vi "报警流程.vi"   [LabVIEW 2016, in "环境动力单元.lvlib"]
uses:
  <vilib>/ptbypt/NI_PtbyPt.lvlib
types:
  T1 = cluster{"低压报警阈值 V":dbl, "低压报警解除阈值 V":dbl, "高温报警阈值 ℃":dbl, "高温报警解除阈值 ℃":dbl, "湿度报警阈值 %":dbl, "湿度报警解除阈值 %":dbl}
  T2 = cluster{"蓄电池电压":dbl, "室温":dbl, "湿度":dbl, "水浸报警":bool, "烟雾报警":bool, "门禁状态":bool}
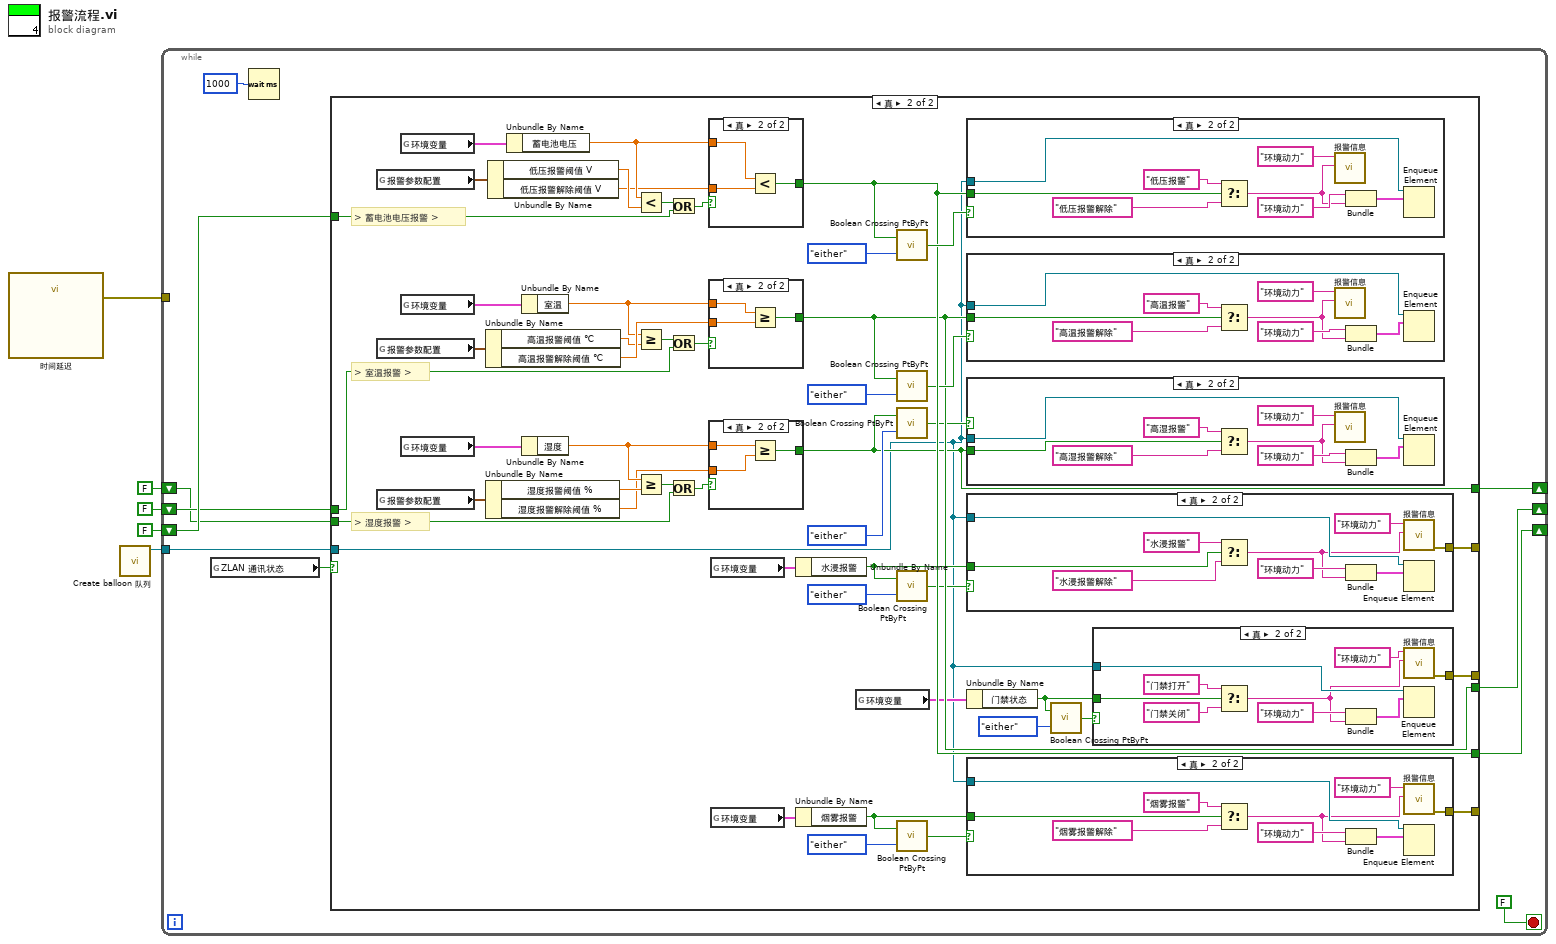
[diagram p0: block diagram]
diagram:
  n1 = call "时间延迟"() -> ("error out"=w1:errorcluster)  [unwired: 11 in]
  n2 = call "Create balloon 队列.vi"() -> ("队列输出"=w5:refnum<queue>)  [unwired: 11 in]
  n3 = while {
    shift-right: [w13] -> _
    shift-left: FALSE -> [w12]
    shift-right: [w10] -> _
    shift-left: FALSE -> [w11]
    shift-right: [w9] -> _
    shift-left: FALSE -> [w8]
    tunnel: w5 -> [w6]
    tunnel: w1 -> [_]
    stop <- FALSE stop-if-true
    n4 = global read "通讯全局变量.vi" "ZLAN 通讯状态"() -> (w7:bool)
    n5 = Wait (ms)(milliseconds to wait=u32 1000 ("等待时间（毫秒）")) -> ()  [unwired: 1 out]
    n6 = case shown="真" w7 {
      tunnel: [_ w38] -> w13
      tunnel: w12 -> [_ w57]
      tunnel: w11 -> [_ w56]
      tunnel: [_ w35] -> w10
      tunnel: [_ w32] -> w9
      tunnel: w8 -> [_ w41]
      tunnel: [_ w27] -> _
      tunnel: [_ w26] -> _
      tunnel: [_ w17] -> _
      tunnel: w6 -> [_ w16]
      frame False {
      }
      frame True {
        # "> 湿度报警 >"
        # "> 室温报警 >"
        # "> 蓄电池电压报警 >"
        n7 = global read "通讯全局变量断电保存.vi" "报警参数配置"() -> (w64:T1)
        n8 = global read "通讯全局变量断电保存.vi" "报警参数配置"() -> (w49:T1)
        n9 = global read "通讯全局变量断电保存.vi" "报警参数配置"() -> (w48:T1)
        n10 = global read "通讯全局变量.vi" "环境变量"() -> (w63:T2)
        n11 = global read "通讯全局变量.vi" "环境变量"() -> (w50:T2)
        n12 = global read "通讯全局变量.vi" "环境变量"() -> (w47:T2)
        n13 = Unbundle By Name(w49) -> ("高温报警阈值 ℃"=w51:dbl, "高温报警解除阈值 ℃"=w54:dbl)
        n14 = Unbundle By Name(w48) -> ("湿度报警阈值 %"=w46:dbl, "湿度报警解除阈值 %"=w43:dbl)
        n15 = Unbundle By Name(w64) -> ("低压报警阈值 V"=w62:dbl, "低压报警解除阈值 V"=w59:dbl)
        n16 = Unbundle By Name(w63) -> ("蓄电池电压"=w60:dbl)
        n17 = Unbundle By Name(w50) -> ("室温"=w53:dbl)
        n18 = Unbundle By Name(w47) -> ("湿度"=w44:dbl)
        n19 = Less?(x=w60, y=w62) -> (x < y?=w61:bool)
        n20 = Greater Or Equal?(x=w53, y=w51) -> (x >= y?=w52:bool)
        n21 = Greater Or Equal?(x=w44, y=w46) -> (x >= y?=w45:bool)
        n22 = Or(x=w61, y=w57) -> (x .or. y?=w58:bool)
        n23 = Or(x=w52, y=w56) -> (x .or. y?=w55:bool)
        n24 = Or(x=w45, y=w41) -> (x .or. y?=w42:bool)
        n25 = case shown="真" w58 {
          tunnel: w60 -> [_ w124]
          tunnel: w59 -> [_ w123]
          tunnel: [_ w122] -> w38
          frame False {
          }
          frame True {
            n26 = Less?(x=w124, y=w123) -> (x < y?=w122:bool)
          }
        }
        n27 = case shown="真" w55 {
          tunnel: w53 -> [_ w121]
          tunnel: w54 -> [_ w120]
          tunnel: [_ w119] -> w35
          frame False {
          }
          frame True {
            n28 = Greater Or Equal?(x=w121, y=w120) -> (x >= y?=w119:bool)
          }
        }
        n29 = case shown="真" w42 {
          tunnel: w44 -> [_ w118]
          tunnel: w43 -> [_ w117]
          tunnel: [_ w116] -> w32
          frame False {
          }
          frame True {
            n30 = Greater Or Equal?(x=w118, y=w117) -> (x >= y?=w116:bool)
          }
        }
        n31 = global read "通讯全局变量.vi" "环境变量"() -> (w29:T2)
        n32 = global read "通讯全局变量.vi" "环境变量"() -> (w24:T2)
        n33 = Unbundle By Name(w29) -> ("水浸报警"=w28:bool)
        n34 = Unbundle By Name(w24) -> ("烟雾报警"=w25:bool)
        n35 = global read "通讯全局变量.vi" "环境变量"() -> (w19:T2)
        n36 = call <vilib>:"Boolean Crossing PtByPt.vi"("direction"=enum16{"either", "false-true", "true-false"}."either", "input"=w38) -> ("crossing"=w39:bool)  [unwired: 1 in]
        n37 = call <vilib>:"Boolean Crossing PtByPt.vi"("direction"=enum16{"either", "false-true", "true-false"}."either", "input"=w35) -> ("crossing"=w36:bool)  [unwired: 1 in]
        n38 = call <vilib>:"Boolean Crossing PtByPt.vi"("direction"=enum16{"either", "false-true", "true-false"}."either", "input"=w32) -> ("crossing"=w34:bool)  [unwired: 1 in]
        n39 = call <vilib>:"Boolean Crossing PtByPt.vi"("direction"=enum16{"either", "false-true", "true-false"}."either", "input"=w28) -> ("crossing"=w30:bool)  [unwired: 1 in]
        n40 = call <vilib>:"Boolean Crossing PtByPt.vi"("direction"=enum16{"either", "false-true", "true-false"}."either", "input"=w25) -> ("crossing"=w23:bool)  [unwired: 1 in]
        n41 = case shown="真" w39 {
          tunnel: w38 -> [_ w114]
          tunnel: w16 -> [_ w109]
          frame False {
          }
          frame True {
            n42 = Select(t="低压报警" ("设备"), s=w114, f="低压报警解除" ("设备")) -> (s? t:f=w108:string)
            n43 = call "报警信息.vi"("报警信息"=w108, "设备"="环境动力") -> ()  [unwired: 9 in, 1 out]
            n44 = Bundle("设备"="环境动力", "设备"=w108) -> (w110:cluster{"设备":string, "设备":string})  [unwired: 1 in]
            n45 = Enqueue Element(queue=w109, element=w110) -> ()  [unwired: 2 in, 3 out]
          }
        }
        n46 = case shown="真" w36 {
          tunnel: w35 -> [_ w106]
          tunnel: w16 -> [_ w101]
          frame False {
          }
          frame True {
            n47 = Select(t="高温报警" ("设备"), s=w106, f="高温报警解除" ("设备")) -> (s? t:f=w100:string)
            n48 = call "报警信息.vi"("报警信息"=w100, "设备"="环境动力") -> ()  [unwired: 9 in, 1 out]
            n49 = Bundle("设备"="环境动力", "设备"=w100) -> (w102:cluster{"设备":string, "设备":string})  [unwired: 1 in]
            n50 = Enqueue Element(queue=w101, element=w102) -> ()  [unwired: 2 in, 3 out]
          }
        }
        n51 = case shown="真" w34 {
          tunnel: w32 -> [_ w98]
          tunnel: w16 -> [_ w93]
          frame False {
          }
          frame True {
            n52 = Select(t="高湿报警" ("设备"), s=w98, f="高湿报警解除" ("设备")) -> (s? t:f=w92:string)
            n53 = call "报警信息.vi"("报警信息"=w92, "设备"="环境动力") -> ()  [unwired: 9 in, 1 out]
            n54 = Bundle("设备"="环境动力", "设备"=w92) -> (w95:cluster{"设备":string, "设备":string})  [unwired: 1 in]
            n55 = Enqueue Element(queue=w93, element=w95) -> ()  [unwired: 2 in, 3 out]
          }
        }
        n56 = case shown="真" w30 {
          tunnel: w28 -> [_ w90]
          tunnel: [_ w87] -> w27
          tunnel: w16 -> [_ w84]
          frame False {
          }
          frame True {
            n57 = Select(t="水浸报警" ("设备"), s=w90, f="水浸报警解除" ("设备")) -> (s? t:f=w83:string)
            n58 = Bundle("设备"="环境动力", "设备"=w83) -> (w86:cluster{"设备":string, "设备":string})  [unwired: 1 in]
            n59 = call "报警信息.vi"("报警信息"=w83, "设备"="环境动力") -> ("error out"=w87:errorcluster)  [unwired: 9 in]
            n60 = Enqueue Element(queue=w84, element=w86) -> ()  [unwired: 2 in, 3 out]
          }
        }
        n61 = Unbundle By Name(w19) -> ("门禁状态"=w18:bool)
        n62 = case shown="真" w23 {
          tunnel: w25 -> [_ w81]
          tunnel: [_ w78] -> w26
          tunnel: w16 -> [_ w77]
          frame False {
          }
          frame True {
            n63 = Select(t="烟雾报警" ("设备"), s=w81, f="烟雾报警解除" ("设备")) -> (s? t:f=w75:string)
            n64 = Bundle("设备"="环境动力", "设备"=w75) -> (w74:cluster{"设备":string, "设备":string})  [unwired: 1 in]
            n65 = call "报警信息.vi"("报警信息"=w75, "设备"="环境动力") -> ("error out"=w78:errorcluster)  [unwired: 9 in]
            n66 = Enqueue Element(queue=w77, element=w74) -> ()  [unwired: 2 in, 3 out]
          }
        }
        n67 = call <vilib>:"Boolean Crossing PtByPt.vi"("direction"=enum16{"either", "false-true", "true-false"}."either", "input"=w18) -> ("crossing"=w20:bool)  [unwired: 1 in]
        n68 = case shown="真" w20 {
          tunnel: w18 -> [_ w72]
          tunnel: [_ w69] -> w17
          tunnel: w16 -> [_ w67]
          frame False {
          }
          frame True {
            n69 = Select(t="门禁打开" ("设备"), s=w72, f="门禁关闭" ("设备")) -> (s? t:f=w66:string)
            n70 = Bundle("设备"="环境动力", "设备"=w66) -> (w65:cluster{"设备":string, "设备":string})  [unwired: 1 in]
            n71 = call "报警信息.vi"("报警信息"=w66, "设备"="环境动力") -> ("error out"=w69:errorcluster)  [unwired: 9 in]
            n72 = Enqueue Element(queue=w67, element=w65) -> ()  [unwired: 2 in, 3 out]
          }
        }
      }
    }
  }
